vi "Intake Height Handler.vi"(11 "JoystickDevRef":T1={"Device"=enum."USB 1"}) -> ()   [LabVIEW 2019]
uses:
  <vilib>/Rock Robotics/WPI/Joystick/WPI_JoystickDevRef.ctl
  <vilib>/Rock Robotics/WPI/Joystick/WPI_JoystickDeviceEnum.ctl
  a2c473c0-4ac3-4127-b44c-c1727d400a3d.vi
panel:
  in  "Setpoint":dbl=39.0 format="%#_13g"
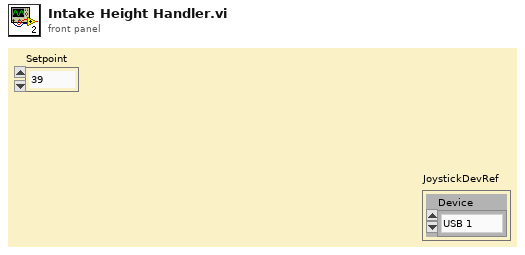
[diagram p1: front panel]
types:
  T1 = typedef "WPI_JoystickDevRef.ctl" = cluster{"Device":T2}
  T2 = typedef "WPI_JoystickDeviceEnum.ctl" = enum16{"USB 0", "USB 1", "USB 2", "USB 3", "USB 4", "USB 5"}
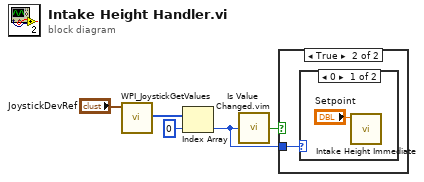
[diagram p0: block diagram]
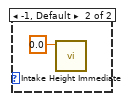
[diagram p3: hidden frame]
diagram:
  n1 = call <vilib>:"WPI_JoystickGetValues.vi"("JoystickDevRef"="JoystickDevRef") -> ("POVs"=w3:i16[])  [unwired: 6 in, 4 out]
  n2 = Index Array(array=w3, index=0) -> (element=w1:i16)
  n3 = call "Is Value Changed.vim"("value"=w1) -> ("changed or first call?"=w2:bool)
  n4 = case shown="True" w2 {
    tunnel: w1 -> [_ w6]
    frame False {
    }
    frame True {
      n5 = case shown="0" w6 {
        frame 0 {
          n6 = call "Intake Height Immediate.vi"("Setpoint"="Setpoint") -> ()  [unwired: 10 in, 1 out]
        }
        frame -1, Default {
          n7 = call "Intake Height Immediate.vi"("Setpoint"=0.0) -> ()  [unwired: 10 in, 1 out]
        }
      }
    }
  }
